vi "Get FileGlobals Prop.vi"(8 "error in (no error)":errorcluster, 11 "SequenceFile in":refnum<class "SequenceFile.lvclass">) -> (0 "error out":errorcluster, 2 "FileGlobals":T1, 3 "SequenceFile out":refnum<class "SequenceFile.lvclass">)   [LabVIEW 2020, in "TSS.lvlib" / "SequenceFile.lvclass"]
uses:
  SequenceFile.lvclass
  VariableContainer/Typedefs/Session Handle.ctl
  VariableContainer/VariableContainer.lvclass
  SequenceFile.lvclass/SequenceFile.ctl
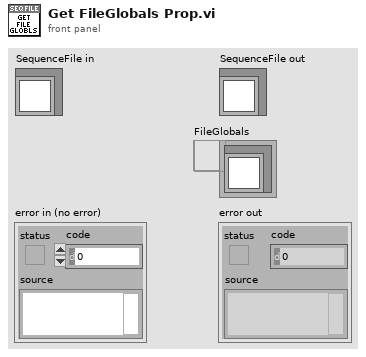
[diagram p1: front panel]
types:
  T1 = typedef "TSS.lvlib/VariableContainer.lvclass/Session Handle.ctl" = refnum<data-value>
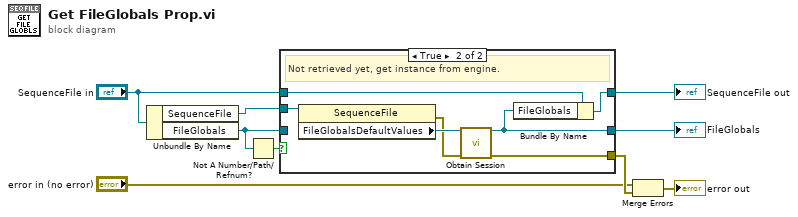
[diagram p0: block diagram]
diagram:
  n1 = Unbundle By Name("SequenceFile in") -> ("SequenceFile"=w8:refnum<k7>, "FileGlobals"=w6:T1)
  n2 = Not A Number/Path/Refnum?(number/path/refnum=w6) -> (NaN/Path/Refnum?=w7:bool)
  n3 = case shown="True" w7 {
    tunnel: w8 -> [_ w18]
    tunnel: [w10 w15] -> w1
    tunnel: w6 -> [w10 _]
    tunnel: "SequenceFile in" -> [w11 w16]
    tunnel: [w11 w14] -> w5
    tunnel: [_ w12] -> w4
    frame False {
      # "Already session'd - simple return"
    }
    frame True {
      # "Not retrieved yet, get instance from engine."
      n4 = property class="SequenceFile"(reference=w18) -> (error out=w13:errorcluster, "FileGlobalsDefaultValues"=w17:refnum<k7>)  [unwired: 1 in, 1 out]
      n5 = call "Obtain Session.vi"("PropertyObject"=w17, "error in (no error)"=w13) -> ("Session Handle"=w15:T1, "error out"=w12:errorcluster)  [unwired: 12 in]
      n6 = Bundle By Name(cluster=w16, "FileGlobals"=w15) -> (w14:refnum<class "SequenceFile.lvclass">)
    }
  }
  "SequenceFile out" <- w5
  "FileGlobals" <- w1
  n7 = Merge Errors("error in (no error)", w4) -> (→"error out":errorcluster)
